vi "Write Library Member Name Replacement.vi"(10 "Library Member Name Replacement":T1, 11 "Project in":refnum<class "Project.lvclass">) -> (3 "Project out":refnum<class "Project.lvclass">)   [LabVIEW 2016, in "Project.lvclass"]
uses:
  Project.lvclass
  Typedefs/LibraryMemberNameReplacement.ctl
  Project.lvclass/Project.ctl
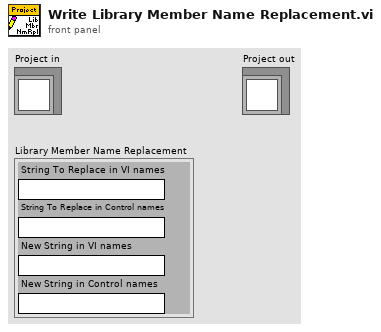
[diagram p1: front panel]
types:
  T1 = typedef "LibraryMemberNameReplacement.ctl" = cluster{"String To Replace in VI names":string, "String To Replace in Control names":string, "New String in VI names":string, "New String in Control names":string}
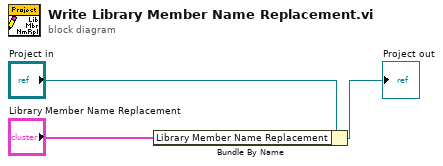
[diagram p0: block diagram]
diagram:
  n1 = Bundle By Name(cluster="Project in", "Library Member Name Replacement"="Library Member Name Replacement") -> (→"Project out":refnum<class "Project.lvclass">)
